vi "Config_LoadKeys.vi"(8 "error in (no error)":errorcluster, 11 "Config In":T3) -> (0 "error out":errorcluster, 2 "output cluster":T1={"General"={"Config.ini"=path "", "Default Logging Path"=path ""}, "Hardware"={"Global T VAR"="", "Global B VAR"="", "VISAS"={"GEN COM"="", "SCOPE COM"="", "VNA COM"=""}}, "Operation"={"Operation Mode"=enum."Idle-Off", "Status"="", "NewLog?"=FALSE, "OvenWarn"=FALSE, "Scope Settings"={"TimeBase"=0.0, "VerticalScale"=4.0}}}, 3 "refnum out":T3)   [LabVIEW 2021]
uses:
  <vilib>/Utility/config.llb/Config Data RefNum.ctl
  Config_Cluster.ctl
  Mode_Enum.ctl
  <vilib>/Utility/config.llb/Read Key (Path).vi
  <vilib>/Utility/config.llb/Read Key (String).vi
  <vilib>/Utility/config.llb/NI_LVConfig.lvlib
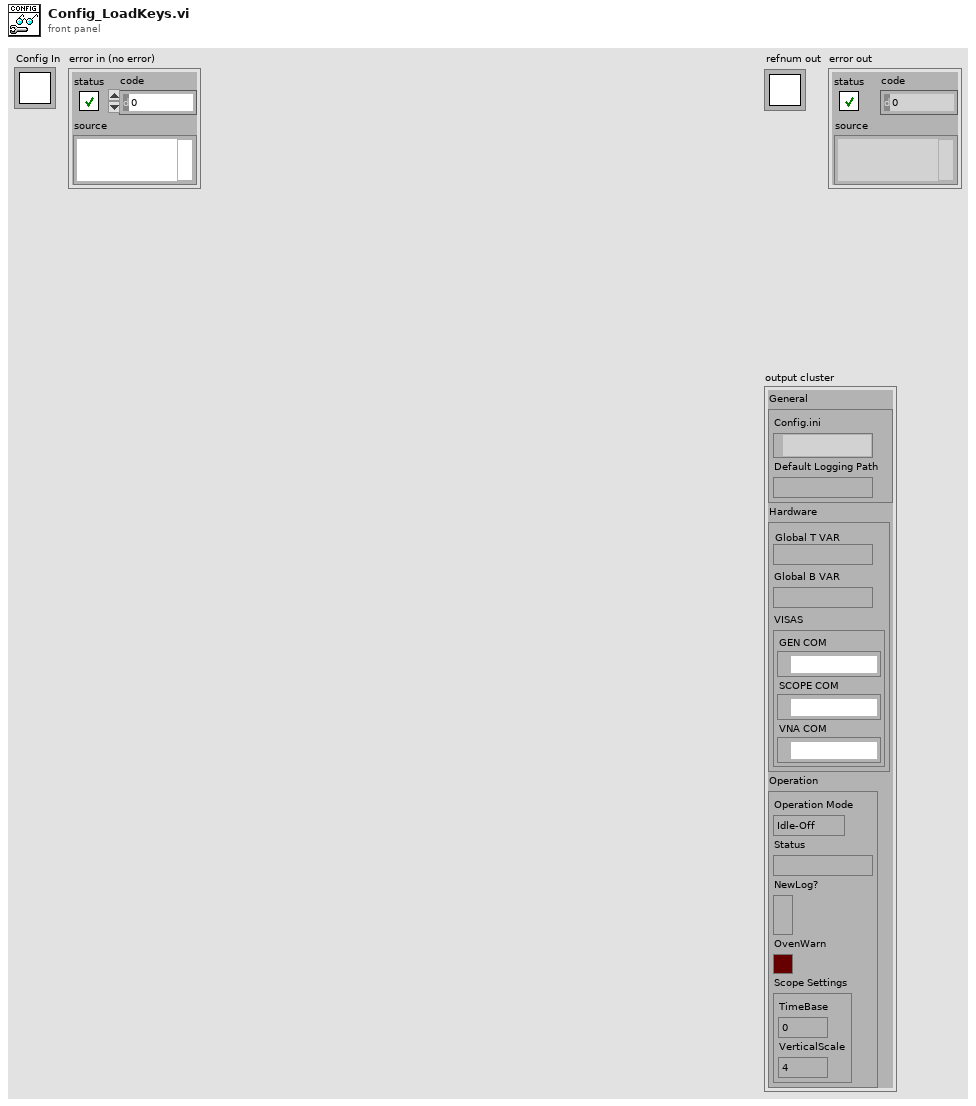
[diagram p1: front panel]
types:
  T1 = typedef "Config_Cluster.ctl" = cluster{"General":cluster{"Config.ini":path, "Default Logging Path":path}, "Hardware":cluster{"Global T VAR":refnum<k21>, "Global B VAR":refnum<k21>, "VISAS":cluster{"GEN COM":refnum<visa-resource-name>, "SCOPE COM":refnum<visa-resource-name>, "VNA COM":refnum<visa-resource-name>}}, "Operation":cluster{"Operation Mode":T2, "Status":string, "NewLog?":bool, "OvenWarn":bool, "Scope Settings":cluster{"TimeBase":dbl, "VerticalScale":dbl}}}
  T2 = typedef "Mode_Enum.ctl" = enum16{"OvenNRDY", "Logging", "Idle-Off", "Idle"}
  T3 = typedef "NI_LVConfig.lvlib/Config Data RefNum.ctl" = refnum<k1>
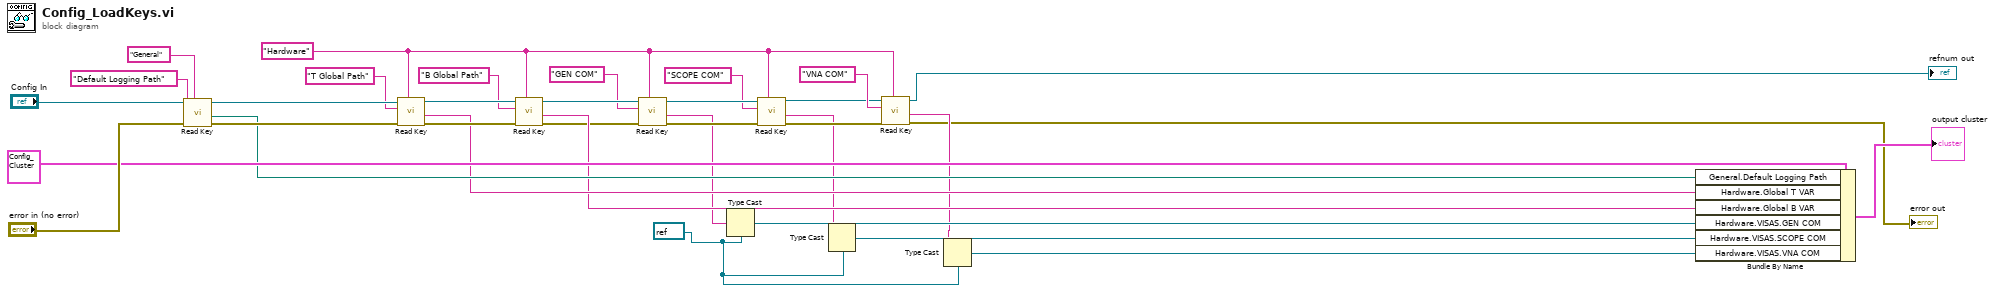
[diagram p0: block diagram]
diagram:
  w5 = refnum<visa-resource-name> refnum ("VISA resource name")
  w10 = "Hardware" ("section")
  n1 = call-poly <vilib>:"Read Key.vi"("section"="General", "error in (no error)"="error in (no error)", "key"="Default Logging Path", "refnum"="Config In") -> ("error out"=w29:errorcluster, "value"=w27:path, "refnum out"=w30:T3)  [unwired: 4 in, 1 out]
  n2 = call-poly <vilib>:"Read Key.vi"("section"=w10, "error in (no error)"=w29, "key"="T Global Path", "refnum"=w30) -> ("error out"=w24:errorcluster, "value"=w21:string, "refnum out"=w25:T3)  [unwired: 4 in, 1 out]
  n3 = call-poly <vilib>:"Read Key.vi"("section"=w10, "error in (no error)"=w24, "key"="B Global Path", "refnum"=w25) -> ("error out"=w18:errorcluster, "value"=w20:string, "refnum out"=w19:T3)  [unwired: 4 in, 1 out]
  n4 = call-poly <vilib>:"Read Key.vi"("section"=w10, "error in (no error)"=w18, "key"="GEN COM", "refnum"=w19) -> ("error out"=w15:errorcluster, "value"=w9:string, "refnum out"=w16:T3)  [unwired: 4 in, 1 out]
  n5 = Type Cast(type=w5, x=w9) -> (*(type *) &x=w8:refnum<visa-resource-name>)
  n6 = call-poly <vilib>:"Read Key.vi"("section"=w10, "error in (no error)"=w15, "key"="SCOPE COM", "refnum"=w16) -> ("error out"=w11:errorcluster, "value"=w4:string, "refnum out"=w12:T3)  [unwired: 4 in, 1 out]
  n7 = Type Cast(type=w5, x=w4) -> (*(type *) &x=w7:refnum<visa-resource-name>)
  n8 = call-poly <vilib>:"Read Key.vi"("section"=w10, "error in (no error)"=w11, "key"="VNA COM", "refnum"=w12) -> ("error out"=→"error out":errorcluster, "value"=w3:string, "refnum out"=→"refnum out":T3)  [unwired: 4 in, 1 out]
  n9 = Type Cast(type=w5, x=w3) -> (*(type *) &x=w6:refnum<visa-resource-name>)
  n10 = Bundle By Name(cluster=T1 {"General"={"Config.ini"=path "", "Default Logging Path"=path ""}, "Hardware"={"Global T VAR"="", "Global B VAR"="", "VISAS"={"GEN COM"="", "SCOPE COM"="", "VNA COM"=""}}, "Operation"={"Operation Mode"=enum."Logging", "Status"="", "NewLog?"=FALSE, "OvenWarn"=FALSE, "Scope Settings"={"TimeBase"=0.0, "VerticalScale"=0.0}}} ("Configuration Cluster"), "General.Default Logging Path"=w27, "Hardware.Global T VAR"=w21, "Hardware.Global B VAR"=w20, "Hardware.VISAS.GEN COM"=w8, "Hardware.VISAS.SCOPE COM"=w7, "Hardware.VISAS.VNA COM"=w6) -> (→"output cluster":T1)
